vi "UpdateOriginList.vi"(7 "Available Points":refnum<vi>, 8 "error in (no error)":errorcluster, 11 "CoordinatteEntry In":T1 {"CaliperSetting"."CaliperEntry"."CaliperType" items=["Distance", "Mid Point", "Perpendicular Projection", "Lines Intersection", "Angle from Horizontal", "Angle from Vertical", "Angle Defined by 3 Points", "Angle Defined by 4 Points", "Bissecting Line", "Mid Line", "Center of Mass", "Area", "Line Fit", "Circle Fit", "Ellipse Fit"]; "OriginPointInfo"."Mode" items=["Horizontal Motion", "Vertical Motion", "Horizontal and Vertical Motion", "Horizontal. Vertical and Angular Motion"]; "AnalysisSetting"."ROI"."Contours"."Type" items=["No Selection", "Point", "Line", "Rectangle", "Oval", "Polygon", "Freehand Region", "Annulus", "Unused2", "Unused3", "Broken Line", "Freehand Line", "Rotated Rectangle"]}) -> (0 "error out":errorcluster, 3 "CoordinatteEntry Out":T1 {"CaliperSetting"."CaliperEntry"."CaliperType" items=["Distance", "Mid Point", "Perpendicular Projection", "Lines Intersection", "Angle from Horizontal", "Angle from Vertical", "Angle Defined by 3 Points", "Angle Defined by 4 Points", "Bissecting Line", "Mid Line", "Center of Mass", "Area", "Line Fit", "Circle Fit", "Ellipse Fit"]; "OriginPointInfo"."Mode" items=["Horizontal Motion", "Vertical Motion", "Horizontal and Vertical Motion", "Horizontal. Vertical and Angular Motion"]; "AnalysisSetting"."ROI"."Contours"."Type" items=["No Selection", "Point", "Line", "Rectangle", "Oval", "Polygon", "Freehand Region", "Annulus", "Unused2", "Unused3", "Broken Line", "Freehand Line", "Rotated Rectangle"]})   [LabVIEW 2019]
uses:
  Control/CoordinatteEntry.ctl
  Process/Controls/Process_Setting.ctl
  Ctrl/VisionProcessName.ctl
  Control/CoordinateAnalysisSetting.ctl
  Control/CoordinateCaliperSetting.ctl
  Caliper/Controls/CaliperDataEntry.ctl
  Caliper/Controls/CaliperType.ctl
  Caliper/Controls/SelectionListEntry.ctl
  Caliper/Controls/SelectionListEntryPointType.ctl
  Caliper/Controls/CaliperResult.ctl
  <vilib>/Utility/miscctls.llb/LVRowAndColumnTypeDef.ctl
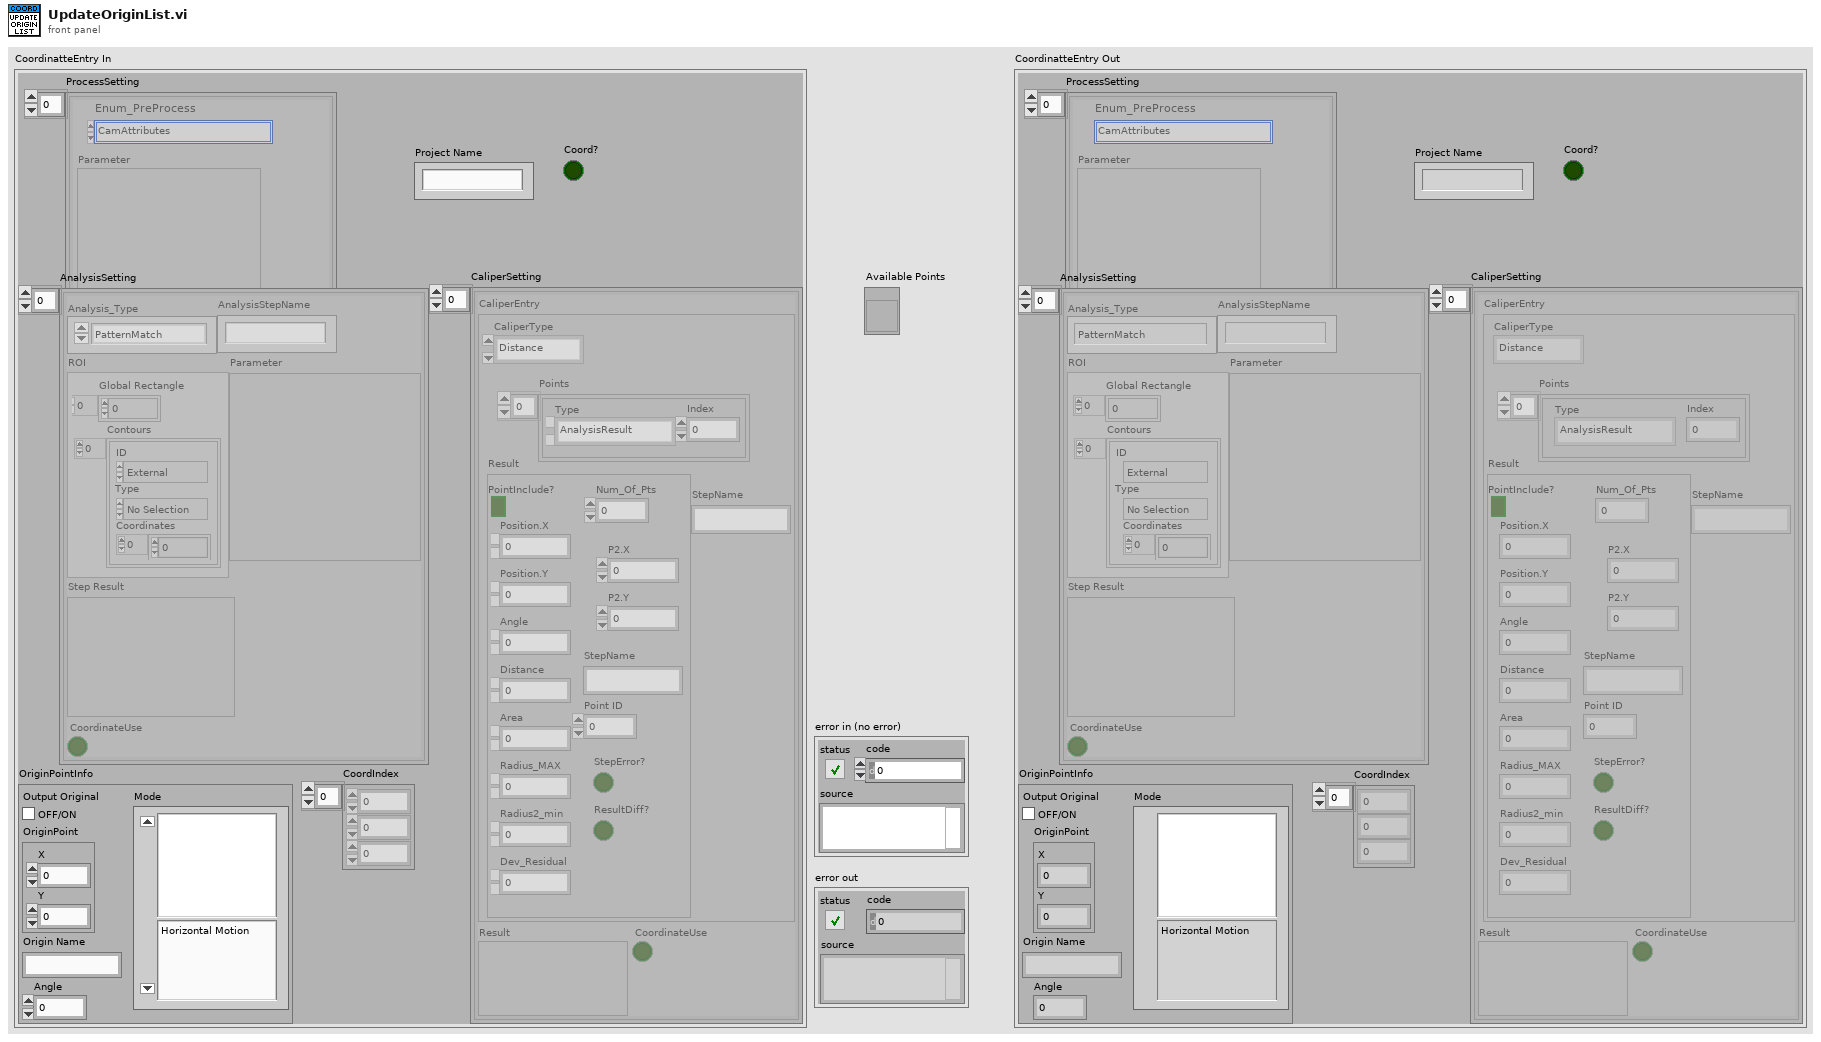
[diagram p1: front panel]
types:
  T1 = typedef "CoordinatteEntry.ctl" = cluster{"ProcessSetting":T2[], "Project Name":string, "AnalysisSetting":T4[], "Coord?":bool, "OriginPointInfo":cluster{"Output Original":bool, "Origin Name":string, "Angle":dbl, "Mode":u16, "OriginPoint":cluster{"X":dbl, "Y":dbl}}, "CaliperSetting":T6[], "CoordIndex":i32[]}
  T2 = typedef "Process_Setting.ctl" = cluster{"Enum_PreProcess":T3, "Parameter":string}
  T3 = typedef "VisionProcessName.ctl" = enum16{"*CamParameter*", "CamAttributes", "*Preprocess*", "CG_Brightness", "C_Plane Extraction", "C_Threshold", "G_Lookup Table", "G_Threshold"}
  T4 = typedef "CoordinateAnalysisSetting.ctl" = cluster{"Analysis_Type":enum16{"PatternMatch", "Straight Edge"}, "ROI ":T5, "Parameter":variant, "Step Result":variant, "AnalysisStepName":string, "CoordinateUse":bool}
  T5 = typedef "ROI Descriptor" = cluster{"Global Rectangle":i32[], "Contours":cluster{"ID":enum32{"External", "Internal"}, "Type":u32, "Coordinates":i32[]}[]}
  T6 = typedef "CoordinateCaliperSetting.ctl" = cluster{"Result":variant, "CoordinateUse":bool, "CaliperEntry":T7}
  T7 = typedef "CaliperDataEntry.ctl" = cluster{"CaliperType":T8, "Points":T9[], "Result":T11, "StepName":string}
  T8 = typedef "CaliperType.ctl" = u32
  T9 = typedef "SelectionListEntry.ctl" = cluster{"Type":T10, "Index":i32}
  T10 = typedef "SelectionListEntryPointType.ctl" = enum16{"AnalysisResult", "CaliperResult"}
  T11 = typedef "CaliperResult.ctl" = cluster{"PointInclude?":bool, "Num_Of_Pts":u8, "Position.X":dbl, "Position.Y":dbl, "Angle":dbl, "Distance":dbl, "Area":dbl, "Radius_MAX":dbl, "Radius2_min":dbl, "Dev_Residual":dbl, "P2.X":dbl, "P2.Y":dbl, "StepName":string, "Point ID":u8, "StepError?":bool, "ResultDiff?":bool}
  T12 = typedef "LVRowAndColumnTypeDef.ctl" = cluster{"Row":i32, "Column":i32}
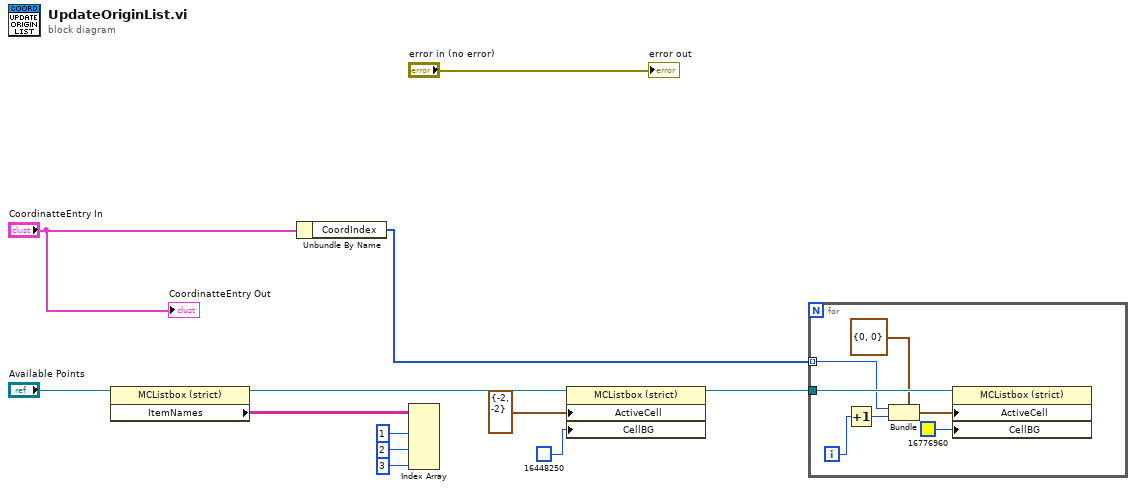
[diagram p0: block diagram]
diagram:
  n1 = property class="MCListbox (strict)"(reference="Available Points") -> (reference out=w4:refnum<vi>, "ItemNames"=w11:string[][])  [unwired: 1 in, 1 out]
  n2 = Unbundle By Name("CoordinatteEntry In") -> ("CoordIndex"=w5:i32[])
  n3 = Index Array(array=w11, index (col) #1=1 ("disabled index (col)"), index (col) #2=2 ("index (col)"), index (col) #3=3 ("index (col)")) -> ()  [unwired: 3 in, 3 out]
  n4 = property class="MCListbox (strict)"(reference=w4, "ActiveCell"=T12 {"Row"=-2, "Column"=-2} ("Active Cell:Active Cell"), "CellBG"=u32 16448250) -> (reference out=w3:refnum<vi>)  [unwired: 1 in, 1 out]
  n5 = for {
    tunnel: w3 -> [w19]
    tunnel: w5 -> [w14] mode=indexing
    i -> [w17]
    n6 = Increment(x=w17) -> (x+1=w16:i32)
    n7 = Bundle(cluster=T12 {"Row"=0, "Column"=0} ("Active Cell:Active Cell"), "Row"=w14, "Column"=w16) -> (w15:T12)
    n8 = property class="MCListbox (strict)"(reference=w19, "ActiveCell"=w15, "CellBG"=u32 16776960) -> ()  [unwired: 1 in, 2 out]
  }
  "CoordinatteEntry Out" <- "CoordinatteEntry In"
  "error out" <- "error in (no error)"
